vi "Unflatten Value.vi"(8 "Error In":errorcluster, 10 "Value":string, 11 "Bool In":refnum<class "Bool.lvclass">) -> (0 "Error Out":errorcluster, 3 "Bool Out":refnum<class "Bool.lvclass">)   [LabVIEW 2020, in "NI_VIAnCFGDataStructure.lvlib" / "Bool.lvclass"]
uses:
  <vilib>/addons/analyzer/VIAnCFGDataStructure/Data Types/Bool/Bool.lvclass
  <vilib>/addons/analyzer/VIAnCFGDataStructure/Data Types/Bool/Bool.lvclass/Bool.ctl
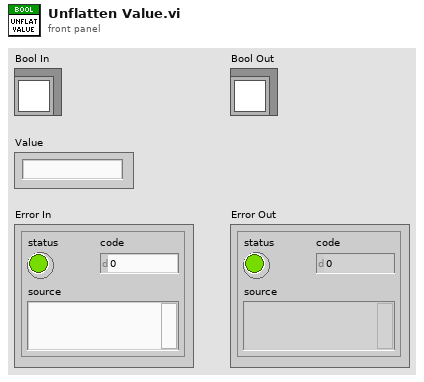
[diagram p1: front panel]
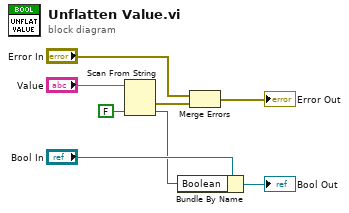
[diagram p0: block diagram]
diagram:
  n1 = Scan From String(input string="Value", default 1=FALSE) -> (error out=w2:errorcluster, output 1=w4:bool)  [unwired: 3 in, 2 out]
  n2 = Bundle By Name(cluster="Bool In", "Boolean"=w4) -> (→"Bool Out":refnum<class "Bool.lvclass">)
  n3 = Merge Errors("Error In", w2) -> (→"Error Out":errorcluster)
